vi "GlobalDeviceList.vi"() -> ()   [LabVIEW 2020]
panel:
  out "设备信息":T1
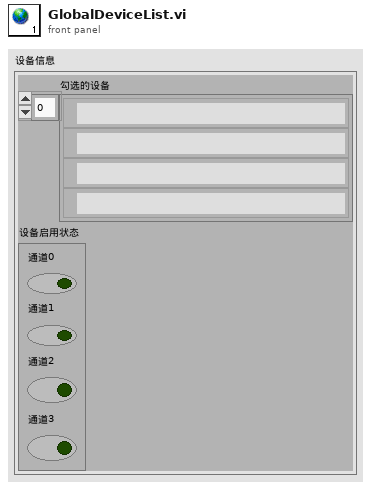
[diagram p1: front panel]
types:
  T1 = cluster{"勾选的设备":refnum<visa-resource-name>[], "设备启用状态":cluster{"通道0":bool, "通道1":bool, "通道2":bool, "通道3":bool}}
diagram:
